vi "ConsigneDebitSimu.vi"() -> ()   [LabVIEW 2012]
panel:
  in  "ConsigneDebitSimu":dbl
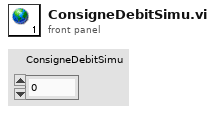
[diagram p1: front panel]
diagram:
